vi "plc time.vi"() -> ()   [LabVIEW 2024]
uses:
  Ctrl/PLC Enum.ctl
  Ctrl/Axis Enum.ctl
panel:
  out "x-y":u32
  out "2deg":u32[](array[numeric])
  out "Array":dbl[](array[numeric])
  in  "step":dbl=80.0 format="%#_13g"
  out "error out":errorcluster caption="错误输出"
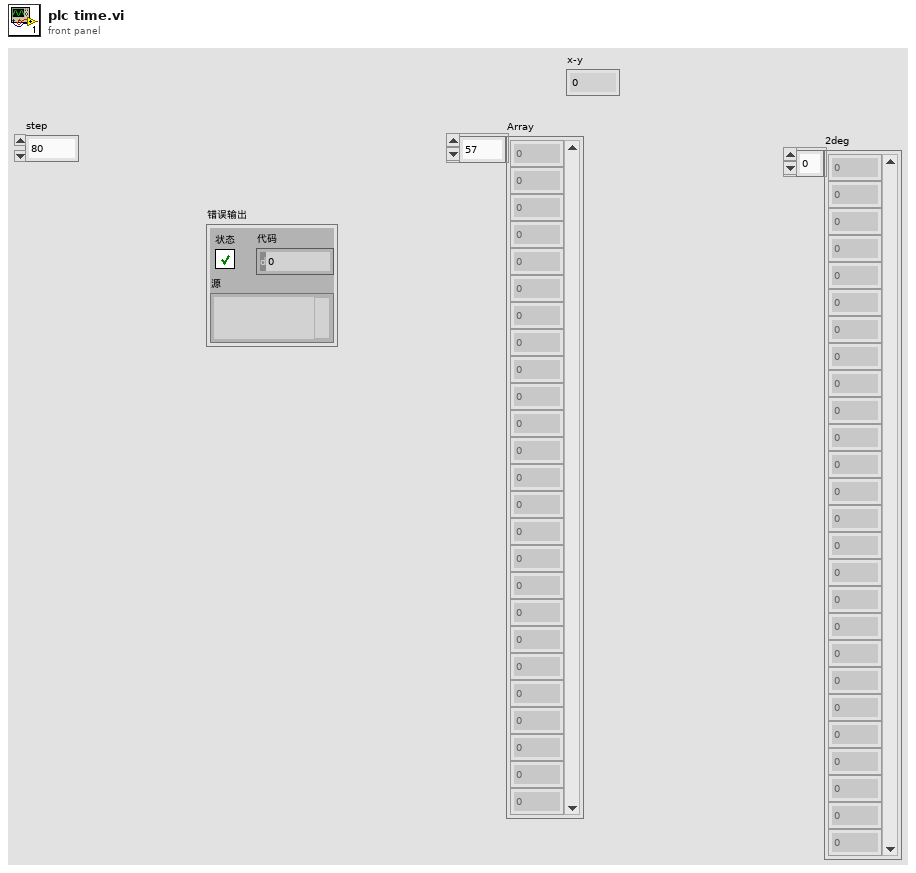
[diagram p1: front panel]
types:
  T1 = typedef "PLC Enum.ctl" = enum16{"Init", "Enable", "Orign", "Load", "Start", "Stop", "StartTest", "StopTest", "Reflector", "WriteResult", "SetSpeed", "SetOrign", "SetLoad", "ServoStatus?", "EquipStatus?", "Origin?", "TestStatus?", "Loadstatus?", "DUTStatus?", "Mes?", "Error？", "Position？", "Speed?", "PinCount", "RunMode", "SN", "Reset", "Jog+", "Jog-", "Close", "Up", "Down", "Clamp", "Release", "In", "Out", "EnterTestMode", "ExitTestMode", "StartButton", "ScanOK", "Power"}
  T2 = typedef "Axis Enum.ctl" = enum16{"Az", "El"}
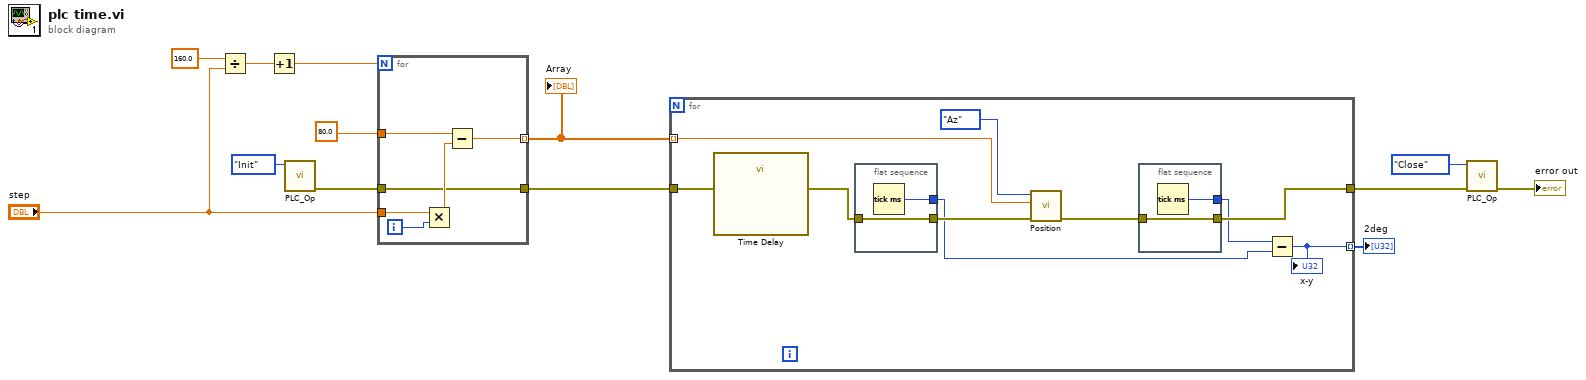
[diagram p0: block diagram]
diagram:
  n1 = Divide(x=160.0, y="step") -> (x/y=w2:dbl)
  n2 = Increment(x=w2) -> (x+1=w1:dbl)
  n3 = call "PLC_Op.vi"("Status"=PLC_Enum."Init") -> ("error out"=w9:errorcluster)  [unwired: 5 in, 5 out]
  n4 = for {
    N: w1 -> [_]
    tunnel: w9 -> [w15]
    tunnel: 80.0 -> [w19]
    tunnel: "step" -> [w17]
    tunnel: [w15] -> w7
    tunnel: [w14] -> w6 mode=indexing
    i -> [w18]
    n5 = Multiply(x=w17, y=w18) -> (x*y=w16:dbl)
    n6 = Subtract(x=w19, y=w16) -> (x-y=w14:dbl)
  }
  "Array" <- w6
  n7 = for {
    tunnel: w7 -> [w27]
    tunnel: [w24] -> w12
    tunnel: w6 -> [w28] mode=indexing
    tunnel: [w21] -> w5 mode=indexing
    n8 = call "Time Delay"("error in (no error)"=w27) -> ("error out"=w20:errorcluster)  [unwired: 10 in]
    n9 = flat-sequence {
      tunnel: w20 -> [w33]
      tunnel: [w33] -> w26
      tunnel: [w32] -> w22
      frame #0 {
        n10 = Tick Count (ms)() -> (millisecond timer value=w32:u32)
      }
    }
    n11 = call "Position.vi"("error in (no error)"=w26, "Position"=w28, "Axis Enum"=Axis_Enum."Az") -> ("error out"=w25:errorcluster)  [unwired: 8 in]
    n12 = flat-sequence {
      tunnel: w25 -> [w31]
      tunnel: [w31] -> w24
      tunnel: [w30] -> w23
      frame #0 {
        n13 = Tick Count (ms)() -> (millisecond timer value=w30:u32)
      }
    }
    n14 = Subtract(x=w23, y=w22) -> (x-y=w21:u32)
    "x-y" <- w21
  }
  "2deg" <- w5
  n15 = call "PLC_Op.vi"("error in (no error)"=w12, "Status"=PLC_Enum."Close") -> ("error out"=→"error out":errorcluster)  [unwired: 4 in, 5 out]
